vi "Create Fast Draw Object.vi"(6 "Actual Transform In":T1, 8 "error in (no error)":errorcluster, 9 "Multiplot Representation In":T3, 10 "3D Ribbon.lvclass in":refnum<class "3D Ribbon.lvclass">, 11 "Plot Object In":refnum<vi>) -> (0 "error out":errorcluster, 1 "Multiplot Representation Out":T3, 2 "3D Ribbon.lvclass out":refnum<class "3D Ribbon.lvclass">, 3 "Plot Object Out":refnum<vi>, 4 "Actual Transform Out":T1)   [LabVIEW 2020, in "3D Ribbon.lvclass"]
uses:
  <vilib>/Math Plots/3D Math Plots/3D Ribbon/3D Ribbon/3D Ribbon.lvclass
  <vilib>/Math Plots/3D Math Plots/3D Plot/3D Plot/Typedef/Multiplot Representation.ctl
  <vilib>/Math Plots/3D Math Plots/3D Plot/3D Plot/Typedef/Plot Representation.ctl
  <vilib>/Math Plots/3D Math Plots/3D Plot/3D Plot/Typedef/Range Clusters.ctl
  <vilib>/Math Plots/3D Math Plots/3D Plot/3D Plot/Typedef/Mesh Data.ctl
  <vilib>/Math Plots/3D Math Plots/3D Plot/3D Plot/Typedef/Actual Transform.ctl
  <vilib>/Math Plots/3D Math Plots/3D Ribbon/3D Ribbon/3D Ribbon.lvclass/3D Ribbon.ctl
  <vilib>/Math Plots/3D Math Plots/3D Plot/3D Plot/3D Plot.lvclass
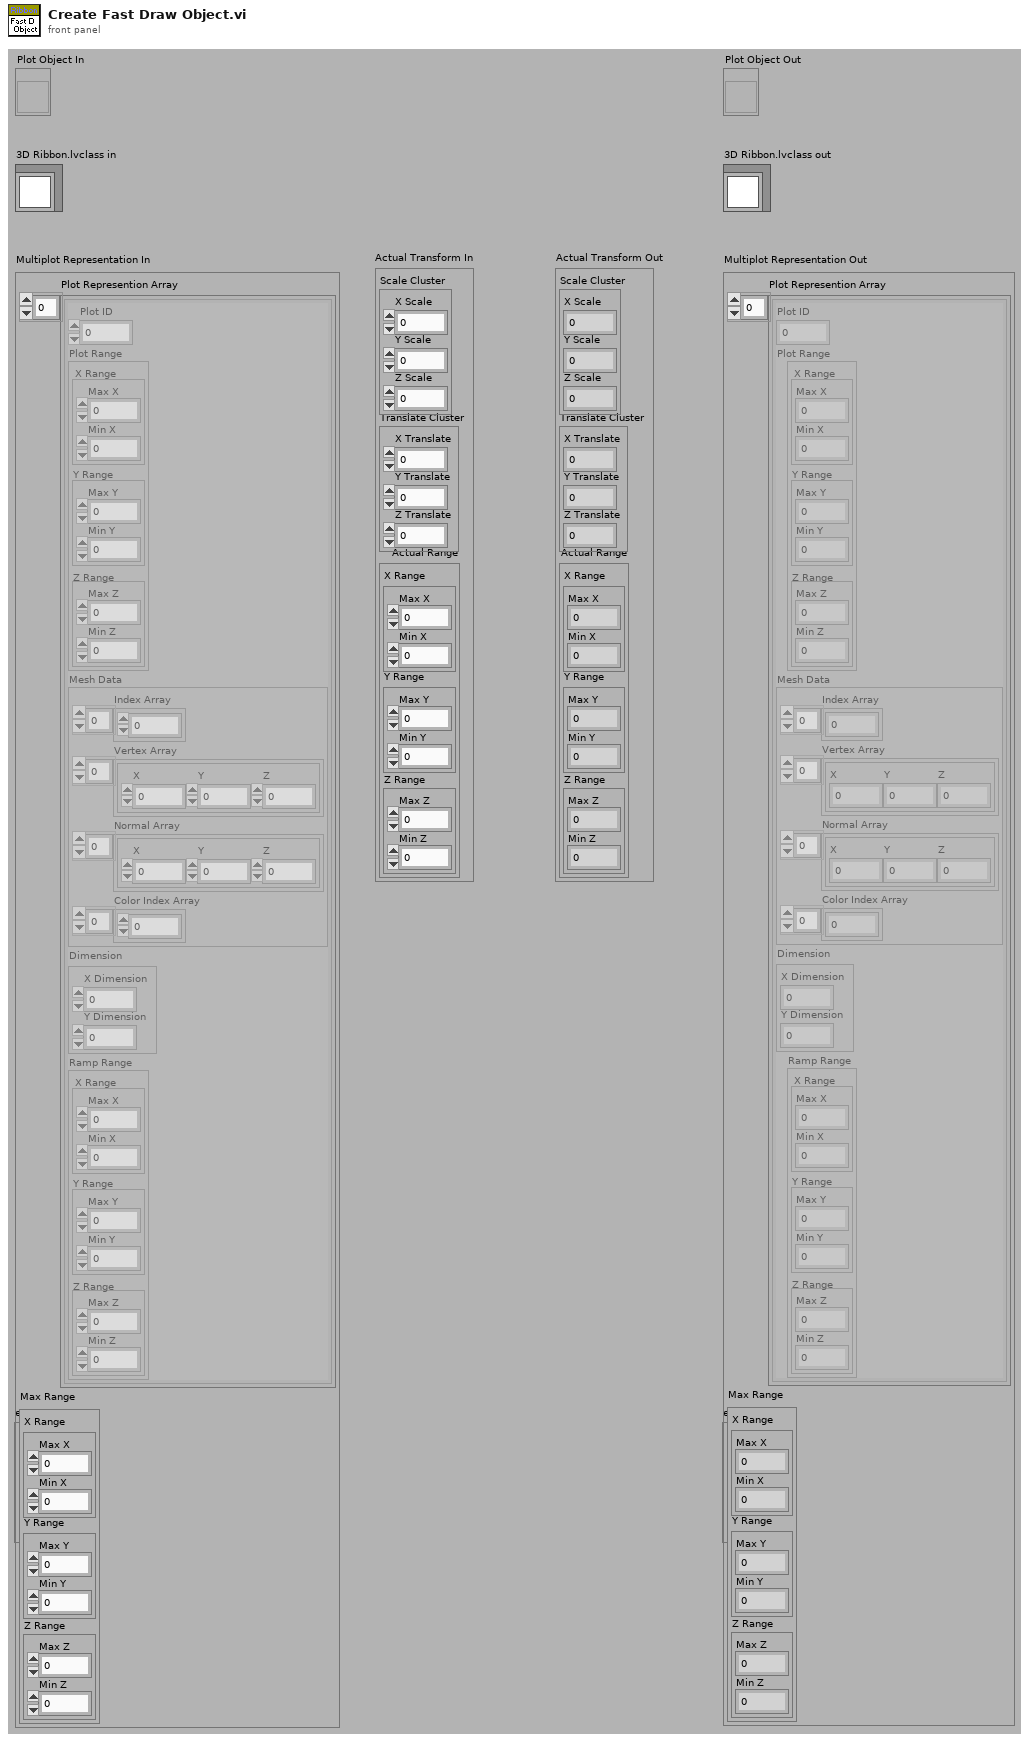
[diagram p1: front panel]
types:
  T1 = typedef "3D Plot.lvclass/Actual Transform.ctl" = cluster{"Scale Cluster":cluster{"X Scale":sgl, "Y Scale":sgl, "Z Scale":sgl}, "Translate Cluster":cluster{"X Translate":sgl, "Y Translate":sgl, "Z Translate":sgl}, "Actual Range":T2}
  T2 = typedef "3D Plot.lvclass/Range Clusters.ctl" = cluster{"X Range":cluster{"Max X":sgl, "Min X":sgl}, "Y Range":cluster{"Max Y":sgl, "Min Y":sgl}, "Z Range":cluster{"Max Z":sgl, "Min Z":sgl}}
  T3 = typedef "3D Plot.lvclass/Multiplot Representation.ctl" = cluster{"Plot Represention Array":T4[], "Max Range":T2}
  T4 = typedef "3D Plot.lvclass/Plot Representation.ctl" = cluster{"Plot ID":i32, "Plot Range":T2, "Mesh Data":T5, "Dimension":cluster{"X Dimension":i32, "Y Dimension":i32}, "Ramp Range":T2}
  T5 = typedef "3D Plot.lvclass/Mesh Data.ctl" = cluster{"Index Array":u32[], "Vertex Array":cluster{"X":sgl, "Y":sgl, "Z":sgl}[], "Normal Array":cluster{"X":sgl, "Y":sgl, "Z":sgl}[], "Color Index Array":i32[]}
  T6 = typedef "3D Ribbon.lvclass/3D Ribbon Property Array.ctl" = T7[]
  T7 = typedef "3D Ribbon.lvclass/3D Ribbon Property.ctl" = cluster{"General Property":cluster{"Plot Name":string, "Coordinate System":enum16{"Cartesian", "Cylindrical", "Spherical"}, "Opacity":sgl}, "Projection Property":cluster{"Draw XY":bool, "Draw YZ":bool, "Draw XZ":bool}, "Plot Property":cluster{"Draw Surface":bool, "Color Ramp Cluster":T8, "Line Style":T9, "Line Width":sgl, "Line Color":u32, "Antialiasing":bool}, "Ribbon Property":cluster{"Ribbon Mode":enum16{"Row", "Column"}, "Ribbon Width":sgl}}
  T8 = typedef "3D Plot.lvclass/Color Ramp Cluster.ctl" = cluster{"Color Ramp Style":enum16{"None", "Shaded", "Color spectrum", "Grey scale", "Custom"}, "Color Ramp Array":u32[], "Color Ramp Index":i32[], "Interpolate?":bool, "Logarithm?":bool}
  T9 = typedef "3D Plot.lvclass/Line Type.ctl" = enum16{"None", "Solid", "Dash", "Dot", "Dash Dot"}
  T10 = enum16{"Points", "Lines", "Line Strip", "Line Loop", "Triangles", "Triangle Strip", "Triangle Fan", "Quads", "Quad Strip", "Polygon"}
  T11 = cluster{"Draw XY":bool, "Draw YZ":bool, "Draw XZ":bool}
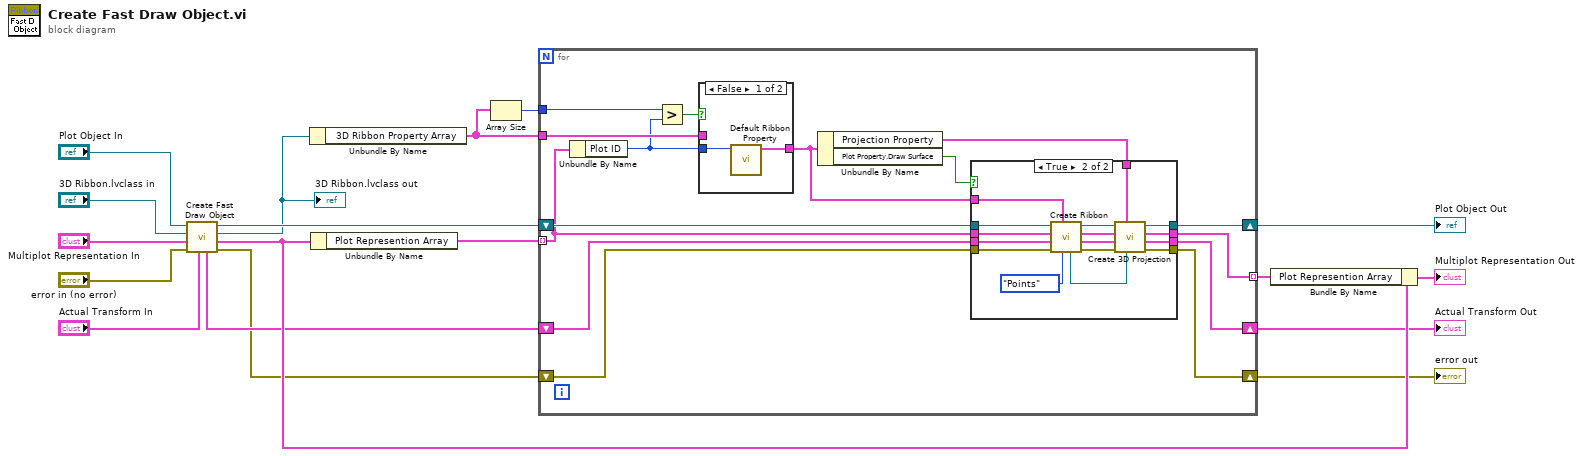
[diagram p0: block diagram]
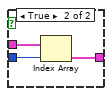
[diagram p3: hidden frame]
diagram:
  n1 = call-parent "Create Fast Draw Object.vi"("Actual Transform In"="Actual Transform In", "error in (no error)"="error in (no error)", "Multiplot Representation In"="Multiplot Representation In", "3D Plot.lvclass in"="3D Ribbon.lvclass in", "Plot Object In"="Plot Object In") -> ("error out"=w4:errorcluster, "Multiplot Representation Out"=w10:T3, "3D Plot.lvclass out"=w3:refnum<class "3D Ribbon.lvclass">, "Plot Object Out"=w11:refnum<vi>, "Actual Transform Out"=w9:T1)  [unwired: 2 out]
  "3D Ribbon.lvclass out" <- w3
  n2 = Unbundle By Name(w3) -> ("3D Ribbon Property Array"=w2:T6)
  n3 = Unbundle By Name(w10) -> ("Plot Represention Array"=w13:T4[])
  n4 = Array Size(array=w2) -> (size(s)=w1:i32)
  n5 = for {
    shift-right: [w30] -> w5
    shift-left: w4 -> [w31]
    shift-right: [w27] -> w7
    shift-left: w11 -> [w33]
    shift-right: [w29] -> w6
    shift-left: w9 -> [w25]
    tunnel: w13 -> [w32] mode=indexing
    tunnel: [w28] -> w12 mode=indexing
    tunnel: w2 -> [w22]
    tunnel: w1 -> [w23]
    n6 = Unbundle By Name(w32) -> ("Plot ID"=w21:i32)
    n7 = Greater?(x=w23, y=w21) -> (0:w24:bool)
    n8 = case shown="False" w24 {
      tunnel: w22 -> [_ w56]
      tunnel: [w52 w55] -> w20
      tunnel: w21 -> [w53 w54]
      frame False {
        n9 = call <vilib>:"Default Ribbon Property.vi"("Plot ID"=w53) -> ("Default Property"=w52:T7)  [unwired: 10 out]
      }
      frame True {
        n10 = Index Array(array=w56, index=w54) -> (element=w55:T7)
      }
    }
    n11 = Unbundle By Name(w20) -> ("Projection Property"=w26:T11, "Plot Property.Draw Surface"=w19:bool)
    n12 = case shown="True" w19 {
      tunnel: w33 -> [w37 w51]
      tunnel: w32 -> [w36 w50]
      tunnel: w31 -> [w34 w49]
      tunnel: [w34 w47] -> w30
      tunnel: [w35 w46] -> w29
      tunnel: [w36 w45] -> w28
      tunnel: [w37 w43] -> w27
      tunnel: w26 -> [_ w41]
      tunnel: w25 -> [w35 w39]
      tunnel: w20 -> [_ w38]
      frame False {
      }
      frame True {
        n13 = call <vilib>:"Create Ribbon.vi"("Draw Mode"=T10."Points", "3D Ribbon Property"=w38, "error in (no error)"=w49, "Plot Representation In"=w50, "Plot Object In"=w51) -> ("error out"=w48:errorcluster, "Plot Representation Out"=w45:T4, "Plot Object Out"=w44:refnum<vi>, "Ribbon Object Out"=w42:refnum<vi>)  [unwired: 1 in, 2 out]
        n14 = call <vilib>:"Create 3D Projection.vi"("Sub Object In"=w42, "Projection Property"=w41, "error in (no error)"=w48, "Actual Transform In"=w39, "Plot Object In"=w44) -> ("error out"=w47:errorcluster, "Actual Transform Out"=w46:T1, "Plot Object Out"=w43:refnum<vi>)  [unwired: 1 in, 3 out]
      }
    }
  }
  "error out" <- w5
  "Plot Object Out" <- w7
  "Actual Transform Out" <- w6
  n15 = Bundle By Name(cluster=w10, "Plot Represention Array"=w12) -> (→"Multiplot Representation Out":T3)
